vi "ExposeMapperGetNamepathAssignableValue.vi"(11 "Data Val Ref in":refnum<data-value>) -> (3 "Data Val Ref Out":refnum<data-value>)   [LabVIEW 2017]
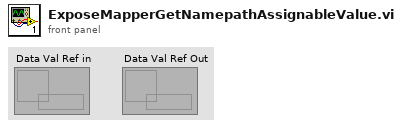
[diagram p1: front panel]
types:
  T1 = typedef "ExposeMapperDataTypeEnum.ctl" = enum16{"NotData", "int8", "byte", "int16", "uint16", "int32", "uint32", "int64", "uint64", "Single", "Double", "String", "Boolean", "Container"}
  T2 = typedef "ExposeObjectMapContainerTypeEnum.ctl" = enum16{"Value", "Array", "Waveform", "NetContainer"}
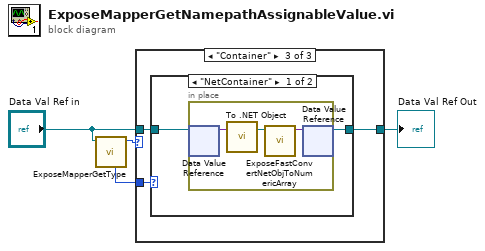
[diagram p0: block diagram]
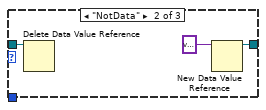
[diagram p3: hidden frame]
diagram:
  n1 = call "ExposeMapperGetType.vi"("Data Val Ref in"="Data Val Ref in") -> ("DataType"=w4:T1, "Container Type (Labview Value type)"=w3:T2)  [unwired: 5 in, 4 out]
  n2 = case shown="\"Container\"" w4 {
    tunnel: [w5 w6 w11] -> w1
    tunnel: w3 -> [_ _ w10]
    tunnel: "Data Val Ref in" -> [w5 w8 w9]
    frame Default {
    }
    frame "NotData" {
      n3 = Delete Data Value Reference(data value reference=w8) -> ()  [unwired: 1 in, 2 out]
      n4 = New Data Value Reference(data value=variant ("Value")) -> (data value reference=w6:refnum<data-value>)  [unwired: 1 in, 1 out]
    }
    frame "Container" {
      n5 = case shown="\"NetContainer\"" w10 {
        tunnel: [w12 w17] -> w11
        tunnel: w9 -> [w13 w17]
        frame "NetContainer" {
          n6 = in-place {
            n7 = in-place-dvr #1(w13) -> (w16:variant)  [unwired: 1 out]
            n8 = call <vilib>:"To .NET Object.vi"("anything"=w16) -> (".NET object"=w15:refnum<k24>)  [unwired: 1 in, 1 out]
            n9 = call "ExposeFastConvertNetObjToNumericArray.vi"(".NET Refnum in"=w15) -> ("Array"=w14:variant)  [unwired: 10 in]
            n10 = in-place-dvr #1(w14) -> (w12:refnum<data-value>)  [unwired: 1 out]
          }
        }
        frame Default {
        }
      }
    }
  }
  "Data Val Ref Out" <- w1
